vi "OBJ_GetHandle.vi"(3 "object name IN":string, 5 "list handle IN":i32) -> (0 "error code OUT":i32, 2 "object handle OUT":i32)   [LabVIEW 2016]
doc: "Retrieves an objects handle.\n\nThis function tries to retrieve an objects handle. This handle is needed for almost every other object related function.\n\nThe functions always needs an object list from where to start the search for the object specified by 'object name IN'. The handle to that list e.g. can be obtained by calling the VI DMR_FindList or any other VI that returns a list handle.\n\nIn some cases a property to be loacted might reside inside a sublist within the specified list.\n\nIn that case the path to that list must be passed as well. Assume that the property 'W' in the sublist 'Aoi' shall be located instead of some property in the root list.\n\nIn that case 'object name IN' must specify the path and name to the property (in this case: 'Aoi/W').\n\nTo find out where to search for a certain property some research work is required, which is done best using the tool 'wxPropView' as it lists all properties the user might need to access in a hierarchical manner. Also the structure of the driver interface might be much easier to understand when looking a this tree structure.\n\nSee also:\nDMR_FindList\n\nThe 'error code OUT' terminal will deliver 0 if successful or a negative error code otherwise. A list of valid error codes and their meaning can be found in the manual about this interface."
uses:
  mvDeviceManager.dll
panel:
  # "OUTPUT"
  # "INPUT"
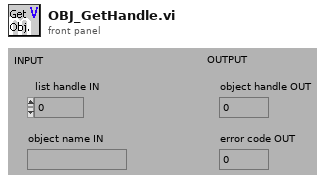
[diagram p1: front panel]
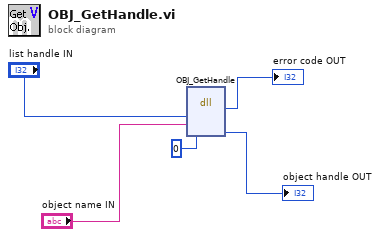
[diagram p0: block diagram]
diagram:
  n1 = dll-call lib="mvDeviceManager.dll" fn="OBJ_GetHandle"("hList"="list handle IN", "pObjectName"="object name IN", "pObjectHandle"=0 ("pListHandle")) -> (→"error code OUT":i32, "pObjectHandle"=→"object handle OUT":i32)  [unwired: 5 in, 2 out]
